vi "TDMS Playback Functional.vi"(1 "Scale Factor Linear":dbl=1.1934598400763813e-07, 4 "IQ Swap Enabled":bool=TRUE, 5 "IQ Rate (S/s)":dbl=25000000.0 format="%#_3p", 6 "pre filter gain":dbl, 7 "channel name (iq/qi)":string="qi", 8 "error in":errorcluster={"status"=FALSE, "code"=373504, "source"="niRFSG Close.vi<ERR>DSP overflow detected. The output waveform was clipped. Reduce the Arb Pre-filter Gain to eliminate overflow."}, 9 "Output Power (dBm)":dbl=10.0 format="%#_3p", 10 "Carrier (Hz)":dbl=3550000000.0 format="%#_3p", 11 "Path":path=path "D:/FOUO/1RDR1P1RDR3.tdms.tdms") -> (0 "error out":errorcluster={"status"=FALSE, "code"=373504, "source"="niRFSG Close.vi<ERR>DSP overflow detected. The output waveform was clipped. Reduce the Arb Pre-filter Gain to eliminate overflow."}, 2 "Playback Progress":i32(slide)=383 scale=-1.0..536.0)   [LabVIEW 2017]
uses:
  <instrlib>/niRFSG/niRFSG.llb/niRFSG Write Arb Waveform (Complex DBL).vi
  MainVI/GlobalVariableS.vi
  <vilib>/FPGAPlugInAG/Dynamic/niLvFpga_Close_Dynamic.vi
  <vilib>/rvi/interface/nirviCloseFPGA/nirviCloseFPGA.xnode
panel:
  out "result string 2":string="3-19-2018"
  in  "input string":string
  out "20 log (scale Factor_Linear)":dbl=-138.46384380841334
  in  "RF:LO Out Enabled":bool
  out "RF:LO Out Power (dBm)":dbl=-0.06505490226659383
  in  "RF:External Gain (dB)":dbl
  in  "RF:Peak Power Adjustment (dB)":dbl
  out "RF:Peak Envelope Power (dBm) =\nPeak Power Adjustment + Output Power":dbl=10.0
  out "RF:Upconverter:Gain (dB)":dbl=4.739916294852831
  out "samples":u32=769639589
  out "number of pending reads 1":u32=8
  out "empty elements":u32=134217728
  out "dma fullness":u32=48764
  out "number of pending reads 2":u32=1
  out "# of elements in host buffer avail for writing":u32=65536
  out "peak fullness":u32
  out "fullness":u32=65536
  out "Completion Loop":i32=3891
  out "fpga peak":u32(slide)=272 scale=-1.0..65536.0
  in  "Monitor Buffer Fullness":bool=TRUE
  out "file peak":u32(slide)=2 scale=0.0..8.0
  out "host peak":u32(slide)=1024 scale=-1.0..134217728.0
  out "File Read Buffer Fullness":u32(slide)=1 scale=0.0..8.0
  out "DMA Host Buffer Emptiness":u32(slide) scale=-1.0..134217728.0
  out "DMA FPGA Buffer Emptiness":u32(slide)=424 scale=-1.0..65536.0
  out "Underflow Detected":bool
  in  "stop button":bool
  in  "Read Block Size (MB)":u32=32 caption="Chunk Size (S)" format="%.0f MB"
  in  "chunks":u32=16 caption="DMA Host Buffer Depth (Blocks)" format="%.0p"
  in  "VST Resource":string="VST"
  # "Config"
  # "Status"
  # "File"
  # "Current"
  # "10/11/2017: +8.57dBm gave -7.23dBm output of the highest peak \n==> Compensate and used Output Power of +8.57+0.24=\n+8.8 dBM to get -7dBm"
  # "Peak"
  # "Current"
  # "Peak"
  # "10/19/2017: +8.8dBm gave -6.44dBm output of the highest peak \n==> Compensate and used Output Power of +8.8-0.47=\n+8.33 dBM to get -7dBm"
  # "RF"
  # "Current"
  # "Peak"
  # "10/19/2017: AutoCal \n==> +8.33 dBm gave -7.22dBm output of the highest peak \n==> Compensate and used Output Power of +8.33+0.22=\n+8.55 dBM to get -7dBm"
  # "Before any other signal processing. \nReduce it to prevent overflow in the AWG interpolation filters. \nSaturates at 7 dB."
  # "After filtering. \nAdjust the output power while keeping the analog path fixed."
  # "Compensate for any Attenuation/Amplification \nbetween Output and DUT"
  # "Refers to PAPR, only used in PEAK Power type.\nIt adds up to Output Power."
  # "20log(1.1534E-6)=  -118.76 dBW\n-118.76 dBW + Correction Factor = -16 dBW \nCorrection Factor = 104.6 dBW"
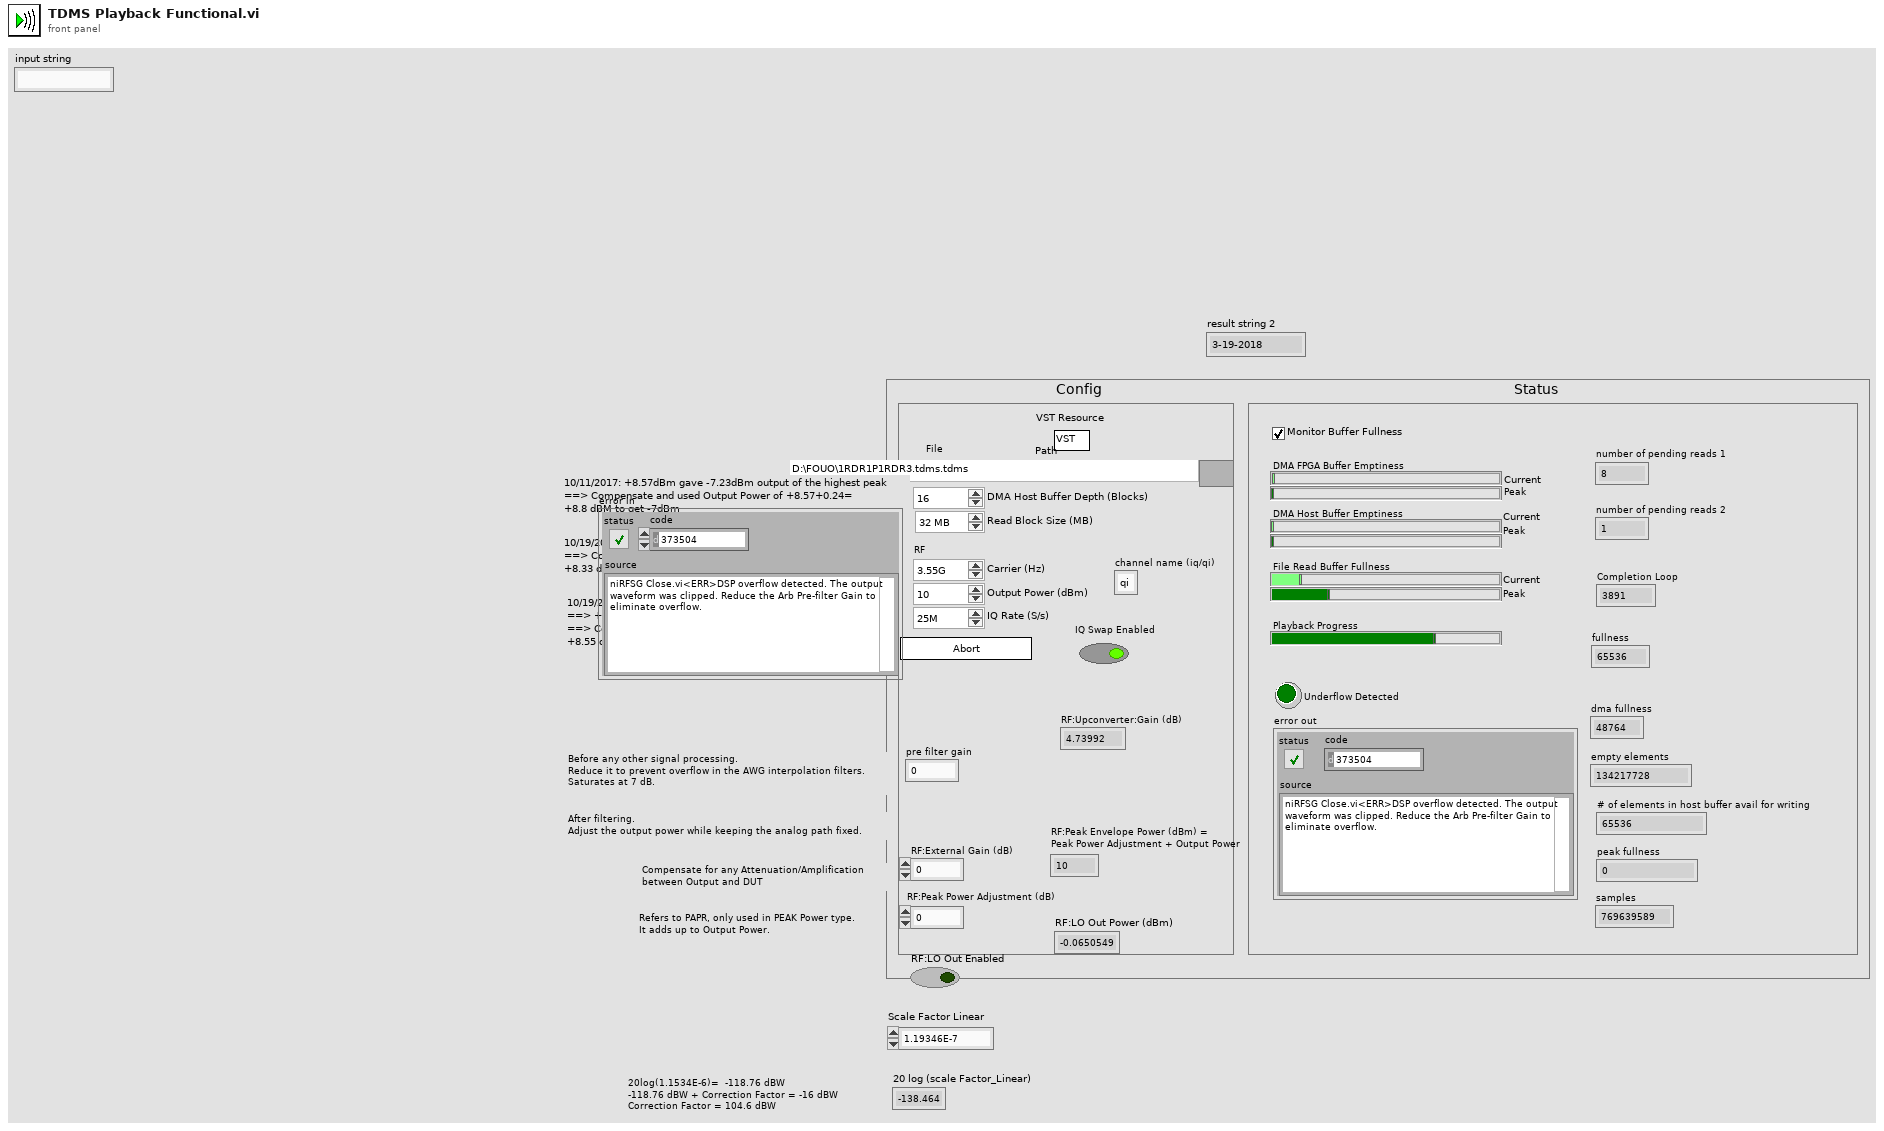
[diagram p1: front panel]
types:
  T1 = enum16{"open", "open or create", "create or replace", "create", "open (read-only)"}
  T2 = cluster{"underflow":bool, "underflows":u32, "samples":u32}
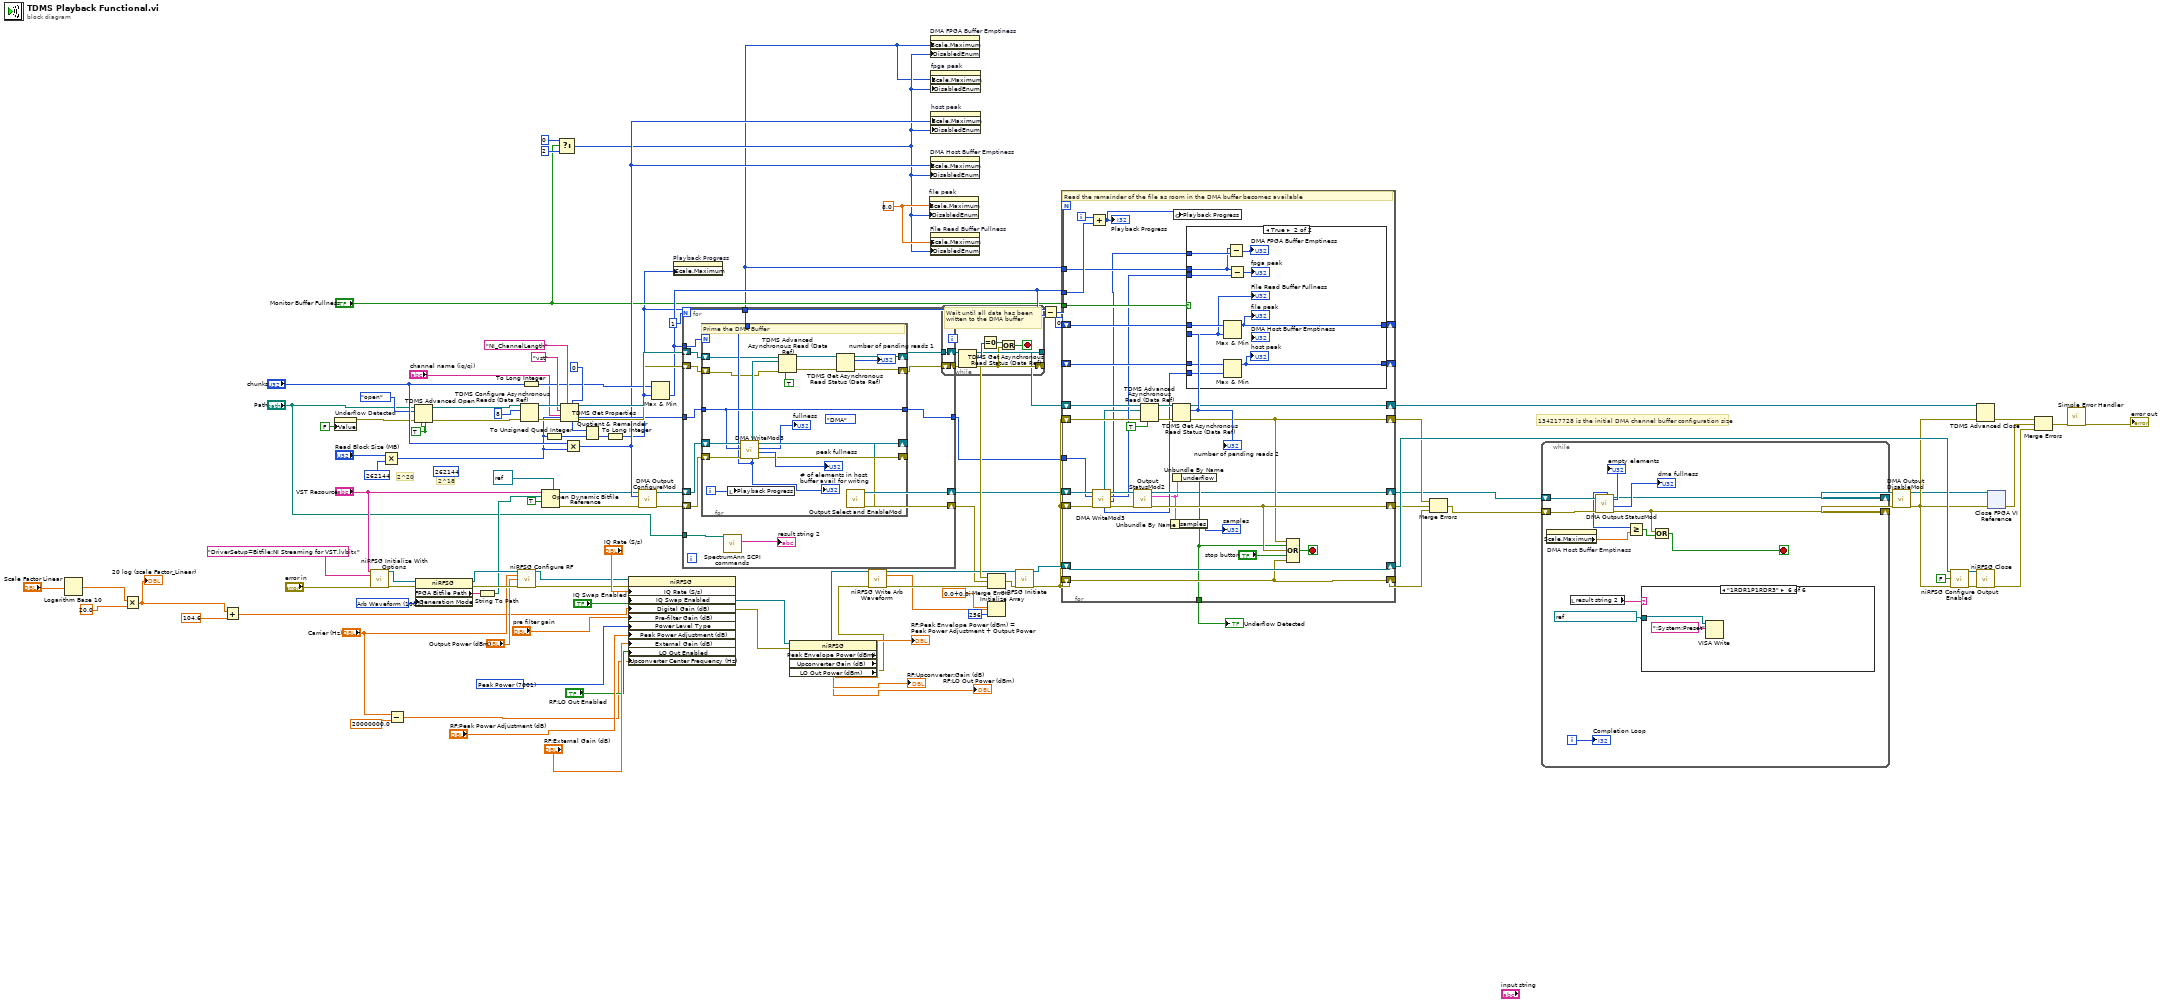
[diagram p0: block diagram]
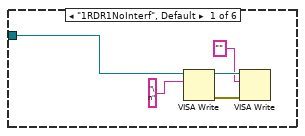
[diagram p3: hidden frame]
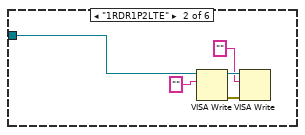
[diagram p4: hidden frame]
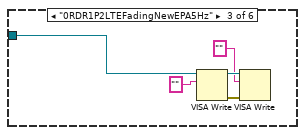
[diagram p5: hidden frame]
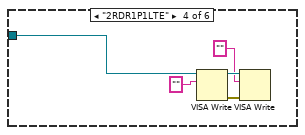
[diagram p6: hidden frame]
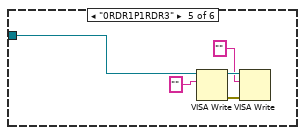
[diagram p7: hidden frame]
diagram:
  w27 = 7001 items=["Average Power"=7000, "Peak Power"=7001] ("RF:Power Level Type")
  (unwired) u32 262144 ("y")
  w51 = 8.0 ("Scale.Range:Maximum")
  w15 = TRUE ("disable buffering? (T)")
  w105 = 1001 items=["CW"=1000, "Arb Waveform"=1001, "Script"=1002] ("Arb:Generation Mode")
  # "134217728 is the initial DMA channel buffer configuration size"
  # "2^20"
  # "2^18"
  n1 = Logarithm Base 10(1:"Scale Factor Linear") -> (0:w9:dbl)
  n2 = Multiply(x=w9, y=20.0) -> (x*y=w8:dbl)
  "20 log (scale Factor_Linear)" <- w8
  n3 = Add(x=w8, y=104.6) -> (x+y=w4:dbl)
  n4 = property on="Underflow Detected" class="Bool (strict)"("Value"=FALSE ("Underflow Detected")) -> (error out=w49:errorcluster)  [unwired: 2 in, 1 out]
  n5 = call <instrlib>:"niRFSG Initialize With Options.vi"("resource name"="VST Resource", "option string"="DriverSetup=Bitfile:NI Streaming for VST.lvbitx", "error in"="error in") -> ("instrument handle"=w110:refnum<k15>, "error out"=w111:errorcluster)  [unwired: 11 in]
  n6 = Multiply(x="Read Block Size (MB)", y=u32 262144) -> (x*y=w59:u32)
  n7 = Subtract(x="Carrier (Hz)", y=20000000.0) -> (x-y=w10:dbl)
  n8 = TDMS Advanced Open(4:w15, 6:w15, 8:w49, 10:T1."open" ("operation (0:open)"), 11:"Path") -> (0:w101:errorcluster, 3:w100:refnum<k34>)  [unwired: 1 out]
  n9 = property class="niRFSG"(reference=w110, error in=w111, "Generation Mode"=w105) -> (reference out=w108:refnum<k15>, error out=w109:errorcluster, "FPGA Bitfile Path"=w107:string)
  n10 = String To Path(string=w107) -> (path=w39:path)
  n11 = call <instrlib>:"niRFSG Configure RF.vi"("instrument handle"=w108, "frequency (Hz)"="Carrier (Hz)", "power level (dBm)"="Output Power (dBm)", "error in"=w109) -> ("instrument handle out"=w26:refnum<k15>, "error out"=w25:errorcluster)  [unwired: 10 in]
  n12 = TDMS Configure Asynchronous Reads (Data Ref)(8:w101, 10:u32 8 ("max asynchronous reads (4)"), 11:w100) -> (0:w90:errorcluster, 3:w91:refnum<k34>)  [unwired: 2 in]
  n13 = To Long Integer(number="chunks") -> (32bit integer=w84:i32)
  n14 = Open Dynamic Bitfile Reference(0:"VST Resource", 1:w39, 2:TRUE ("Run When Loaded"), 4:refnum<k20> refnum ("Type")) -> (5:w30:refnum<k20>, 8:w29:errorcluster)  [unwired: 1 in]
  n15 = To Unsigned Quad Integer(1:w59) -> (0:w62:u64)
  n16 = Select(t=0, s="Monitor Buffer Fullness", f=2) -> (s? t:f=w45:i32)
  n17 = TDMS Get Properties(5:u64 0, 7:"NI_ChannelLength" ("property name"), 8:w90, 9:"channel name (iq/qi)", 10:"vst" ("group name"), 11:w91) -> (0:w88:errorcluster, 3:w89:refnum<k34>, 4:w67:u64)  [unwired: 3 out]
  n18 = Multiply(x="chunks", y=w59) -> (x*y=w57:u32)
  n19 = Quotient & Remainder(x=w67, y=w62) -> (floor(x/y)=w66:u64)  [unwired: 1 out]
  n20 = To Long Integer(number=w66) -> (32bit integer=w52:i32)
  n21 = property class="niRFSG"(reference=w26, error in=w25, "IQ Rate (S/s)"="IQ Rate (S/s)", "IQ Swap Enabled"="IQ Swap Enabled", "Digital Gain (dB)"=w4, "Pre-filter Gain (dB)"="pre filter gain", "Power Level Type"=w27, "Peak Power Adjustment (dB)"="RF:Peak Power Adjustment (dB)", "External Gain (dB)"="RF:External Gain (dB)", "LO Out Enabled"="RF:LO Out Enabled", "Upconverter Center Frequency (Hz)"=w10) -> (reference out=w22:refnum<k15>, error out=w20:errorcluster)
  n22 = call "DMA Output ConfigureMod.vi"("error in (no error)"=w29, "depth"=w57, "Refnum in"=w30) -> ("error out"=w47:errorcluster, "Refnum out"=w46:refnum<k20>)  [unwired: 7 in]
  n23 = Max & Min(x=w84, y=w52) -> (min(x,y)=w61:i32)  [unwired: 1 out]
  n24 = property on="Playback Progress" class="Slide (strict)"("Scale.Maximum"=w52) -> ()  [unwired: 2 in, 2 out]
  n25 = for {
    N: 1 -> [_]
    tunnel: w61 -> [w124]
    tunnel: w59 -> [w123]
    tunnel: [w119] -> w44
    tunnel: [w117] -> w38
    shift-right: [w128] -> w99
    shift-left: w89 -> [w126]
    shift-right: [w127] -> w98
    shift-left: w88 -> [w125]
    shift-right: [w122] -> w48
    shift-left: w47 -> [w121]
    shift-right: [w118] -> w41
    shift-left: w46 -> [w120]
    tunnel: "Path" -> [w113]
    n26 = for {
      N: w124 -> [_]
      shift-right: [w133] -> w127
      shift-left: w125 -> [w129]
      shift-right: [w136] -> w116
      shift-left: w121 -> [w145]
      shift-right: [w132] -> w128
      shift-left: w126 -> [w130]
      shift-right: [w144] -> w115
      shift-left: w120 -> [w146]
      tunnel: w123 -> [w143]
      tunnel: [w143] -> w117
      tunnel: [w141] -> w119
      i -> [w142]
      (unwired) enum16{"none", "DMA", "local", "P2P", "DIO"}."DMA" ("stream select")
      # "Prime the DMA Buffer"
      n27 = local write "Playback Progress"(w142) -> ()
      n28 = call "DMA WriteMod3.vi"("error in (no error)"=w145, "number of elements"=w143, "Refnum in"=w146) -> ("error out"=w136:errorcluster, "peak fullness"=→"peak fullness":u32, "fullness"=→"fullness":u32, "Refnum out"=w144:refnum<k20>, "empty elements remaining"=w141:u32, "Write Region Reference"=w140:refnum<data-value>)  [unwired: 3 in]
      "# of elements in host buffer avail for writing" <- w141
      n29 = TDMS Advanced Asynchronous Read (Data Ref)(6:TRUE ("auto delete reference? (T)"), 8:w129, 10:w140, 11:w130) -> (0:w134:errorcluster, 3:w135:refnum<k34>)  [unwired: 1 out]
      n30 = TDMS Get Asynchronous Read Status (Data Ref)(8:w134, 11:w135) -> (0:w133:errorcluster, 2:→"number of pending reads 1":u32, 3:w132:refnum<k34>)
    }
    n31 = call "SpectrumAnn SCPI commands.vi"("Path"=w113) -> ("result string"=→"result string 2":string)  [unwired: 8 in, 2 out]
    n32 = call "Output Select and EnableMod.vi"("error in (no error)"=w116, "Refnum in"=w115) -> ("error out"=w122:errorcluster, "Refnum out"=w118:refnum<k20>)  [unwired: 8 in]
  }
  n33 = property class="niRFSG"(reference=w22, error in=w20) -> (reference out=w21:refnum<k15>, error out=w19:errorcluster, "Peak Envelope Power (dBm)"=→"RF:Peak Envelope Power (dBm) =\nPeak Power Adjustment + Output Power":dbl, "Upconverter Gain (dB)"=→"RF:Upconverter:Gain (dB)":dbl, "LO Out Power (dBm)"=→"RF:LO Out Power (dBm)":dbl)
  n34 = property on="file peak" class="Slide (strict)"("Scale.Maximum"=w51, "DisabledEnum"=w45) -> ()  [unwired: 2 in, 2 out]
  n35 = property on="DMA FPGA Buffer Emptiness" class="Slide (strict)"("Scale.Maximum"=w44, "DisabledEnum"=w45) -> ()  [unwired: 2 in, 2 out]
  n36 = property on="DMA Host Buffer Emptiness" class="Slide (strict)"("Scale.Maximum"=w57, "DisabledEnum"=w45) -> ()  [unwired: 2 in, 2 out]
  n37 = property on="File Read Buffer Fullness" class="Slide (strict)"("Scale.Maximum"=w51, "DisabledEnum"=w45) -> ()  [unwired: 2 in, 2 out]
  n38 = property on="fpga peak" class="Slide (strict)"("Scale.Maximum"=w44, "DisabledEnum"=w45) -> ()  [unwired: 2 in, 2 out]
  n39 = property on="host peak" class="Slide (strict)"("Scale.Maximum"=w57, "DisabledEnum"=w45) -> ()  [unwired: 2 in, 2 out]
  n40 = while {
    tunnel: w99 -> [w152]
    shift-right: [w148] -> w95
    shift-left: w98 -> [w153]
    tunnel: [w150] -> w94
    stop <- w149 stop-if-true
    # "Wait until all data has been written to the DMA buffer"
    n41 = TDMS Get Asynchronous Read Status (Data Ref)(8:w153, 11:w152) -> (0:w148:errorcluster, 2:w151:u32, 3:w150:refnum<k34>)
    n42 = Equal To 0?(x=w151) -> (x = 0?=w147:bool)
    n43 = Or(x=w147, y=w148) -> (x .or. y?=w149:bool)
  }
  n44 = Initialize Array(cdb 0.0+0.0i ("element"), 256 ("dimension size")) -> (w35:cdb[])
  n45 = call-poly <instrlib>:"niRFSG Write Arb Waveform.vi"("instrument handle"=w21, "waveform data"=w35, "error in"=w19) -> ("instrument handle out"=w82:refnum<k15>, "error out"=w81:errorcluster)  [unwired: 11 in]
  n46 = Merge Errors(w95, w48, w81) -> (w97:errorcluster)
  n47 = call <instrlib>:"niRFSG Initiate.vi"("instrument handle"=w82, "error in"=w97) -> ("instrument handle out"=w96:refnum<k15>, "error out"=w83:errorcluster)  [unwired: 12 in]
  n48 = Subtract(x=w52, y=w61) -> (x-y=w60:i32)
  n49 = for {
    N: w60 -> [_]
    shift-right: [w187] -> w70
    shift-left: w83 -> [w187]
    shift-right: [w168] -> w71
    shift-left: w83 -> [w175]
    shift-right: [w171] -> w72
    shift-left: w83 -> [w176]
    shift-right: [w167] -> w92
    shift-left: w94 -> [w174]
    shift-right: [w188] -> w78
    shift-left: w96 -> [w188]
    tunnel: w61 -> [w184]
    tunnel: w38 -> [w161]
    tunnel: [w165] -> w58
    shift-right: [w181] -> _
    shift-left: u32 0 -> [w180]
    shift-right: [w179] -> _
    shift-left: _ -> [w178]
    tunnel: "Monitor Buffer Fullness" -> [w177]
    tunnel: w44 -> [w164]
    shift-right: [w160] -> w40
    shift-left: w41 -> [w162]
    i -> [w183]
    stop <- w185 stop-if-true
    # "Read the remainder of the file as room in the DMA buffer becomes available"
    n50 = Add(x=w183, y=w184) -> (x+y=w154:i32)
    "Playback Progress" <- w154
    n51 = call "DMA WriteMod3.vi"("error in (no error)"=w176, "number of elements"=w161, "Refnum in"=w162) -> ("error out"=w172:errorcluster, "peak fullness"=w157:u32, "fullness"=w166:u32, "Refnum out"=w173:refnum<k20>, "empty elements remaining"=w159:u32, "Write Region Reference"=w158:refnum<data-value>)  [unwired: 3 in]
    n52 = call "Output StatusMod2.vi"("error in (no error)"=w172, "Refnum in"=w173) -> ("error out"=w171:errorcluster, "status"=w156:T2, "Refnum out"=w160:refnum<k20>)  [unwired: 7 in]
    n53 = TDMS Advanced Asynchronous Read (Data Ref)(6:TRUE ("auto delete reference? (T)"), 8:w175, 10:w158, 11:w174) -> (0:w170:errorcluster, 3:w169:refnum<k34>)  [unwired: 1 out]
    n54 = Unbundle By Name(w156) -> ("samples"=→"samples":u32)
    n55 = TDMS Get Asynchronous Read Status (Data Ref)(8:w170, 11:w169) -> (0:w168:errorcluster, 2:w182:u32, 3:w167:refnum<k34>)
    "number of pending reads 2" <- w182
    n56 = Unbundle By Name(w156) -> ("underflow"=w165:bool)
    n57 = global write "GlobalVariableS.vi" "Playback Progress"(w154) -> ()
    n58 = case shown="True" w177 {
      tunnel: w182 -> [_ w198]
      tunnel: [_ w196] -> w181
      tunnel: w180 -> [_ w199]
      tunnel: [_ w195] -> w179
      tunnel: w178 -> [_ w197]
      tunnel: w157 -> [_ w191]
      tunnel: w166 -> [_ w193]
      tunnel: w159 -> [_ w194]
      tunnel: w164 -> [_ w190]
      frame False {
      }
      frame True {
        n59 = Max & Min(x=w199, y=w198) -> (max(x,y)=w196:u32)  [unwired: 1 out]
        "file peak" <- w196
        n60 = Max & Min(x=w197, y=w194) -> (max(x,y)=w195:u32)  [unwired: 1 out]
        "host peak" <- w195
        n61 = Subtract(x=w190, y=w191) -> (x-y=→"DMA FPGA Buffer Emptiness":u32)
        n62 = Subtract(x=w190, y=w193) -> (x-y=→"fpga peak":u32)
        "File Read Buffer Fullness" <- w198
      }
    }
    n63 = Compound Arithmetic op=OR(w168, w165, w171, "stop button", w187) -> (w185:bool)
  }
  "Underflow Detected" <- w58
  n64 = Merge Errors(w71, w72, w70) -> (w93:errorcluster)
  n65 = while {
    shift-right: [w207] -> w80
    shift-left: w93 -> [w211]
    shift-right: [w202] -> w79
    shift-left: w40 -> [w210]
    i -> [w209]
    stop <- w208 stop-if-true
    n66 = property on="DMA Host Buffer Emptiness" class="Slide (strict)"() -> ("Scale.Maximum"=w203:dbl)  [unwired: 2 in, 2 out]
    n67 = local read "result string 2"() -> (w200:string)
    n68 = call "DMA Output StatusMod.vi"("error in (no error)"=w211, "Refnum in"=w210) -> ("error out"=w207:errorcluster, "dma fullness"=→"dma fullness":u32, "Refnum out"=w202:refnum<k20>, "empty elements"=w204:u32)  [unwired: 5 in, 1 out]
    "empty elements" <- w204
    n69 = Greater Or Equal?(x=w204, y=w203) -> (x >= y?=w206:bool)
    n70 = case shown="\"1RDR1P1RDR3\"" w200 {
      tunnel: refnum<visa-resource-name> "SpecAnn-9010A-20100" ("VISA resource name") -> [w212 w217 w222 w227 w232 w238]
      frame "1RDR1NoInterf", Default {
        n71 = VISA Write(VISA resource name=w212, write buffer="\n") -> (VISA resource name out=w215:refnum<visa-resource-name>, error out=w214:errorcluster)  [unwired: 1 in, 1 out]
        n72 = VISA Write(VISA resource name=w215, write buffer="", error in (no error)=w214) -> ()  [unwired: 3 out]
      }
      frame "1RDR1P2LTE" {
        n73 = VISA Write(VISA resource name=w217, write buffer="") -> (VISA resource name out=w220:refnum<visa-resource-name>, error out=w219:errorcluster)  [unwired: 1 in, 1 out]
        n74 = VISA Write(VISA resource name=w220, write buffer="", error in (no error)=w219) -> ()  [unwired: 3 out]
      }
      frame "0RDR1P2LTEFadingNewEPA5Hz" {
        n75 = VISA Write(VISA resource name=w222, write buffer="") -> (VISA resource name out=w225:refnum<visa-resource-name>, error out=w224:errorcluster)  [unwired: 1 in, 1 out]
        n76 = VISA Write(VISA resource name=w225, write buffer="", error in (no error)=w224) -> ()  [unwired: 3 out]
      }
      frame "2RDR1P1LTE" {
        n77 = VISA Write(VISA resource name=w227, write buffer="") -> (VISA resource name out=w230:refnum<visa-resource-name>, error out=w229:errorcluster)  [unwired: 1 in, 1 out]
        n78 = VISA Write(VISA resource name=w230, write buffer="", error in (no error)=w229) -> ()  [unwired: 3 out]
      }
      frame "0RDR1P1RDR3" {
        n79 = VISA Write(VISA resource name=w232, write buffer="") -> (VISA resource name out=w235:refnum<visa-resource-name>, error out=w234:errorcluster)  [unwired: 1 in, 1 out]
        n80 = VISA Write(VISA resource name=w235, write buffer="", error in (no error)=w234) -> ()  [unwired: 3 out]
      }
      frame "1RDR1P1RDR3" {
        n81 = VISA Write(VISA resource name=w238, write buffer=":System:Preset") -> ()  [unwired: 1 in, 3 out]
      }
    }
    n82 = Compound Arithmetic op=OR(w207, w206) -> (w208:bool)
    "Completion Loop" <- w209
  }
  n83 = call "DMA Output DisableMod.vi"("error in (no error)"=w80, "Refnum in"=w79) -> ("error out"=w32:errorcluster, "Refnum out"=w31:refnum<k20>)  [unwired: 8 in]
  n84 = call <instrlib>:"niRFSG Configure Output Enabled.vi"("instrument handle"=w78, "output enabled"=FALSE, "error in"=w32) -> ("instrument handle out"=w76:refnum<k15>, "error out"=w77:errorcluster)  [unwired: 11 in]
  n85 = TDMS Advanced Close(8:w32, 11:w92) -> (0:w65:errorcluster)  [unwired: 2 in, 1 out]
  n86 = call <instrlib>:"niRFSG Close.vi"("instrument handle"=w76, "error in"=w77) -> ("error out"=w63:errorcluster)  [unwired: 13 in]
  n87 = xnode "Close FPGA VI Reference"("FPGA VI Reference In"=w31, "error in"=w32) -> ("error out"=w64:errorcluster)
  n88 = Merge Errors(w65, w64, w63) -> (w33:errorcluster)
  "error out" <- w33
  n89 = call <vilib>:"Simple Error Handler.vi"("error in (no error)"=w33) -> ()  [unwired: 4 in, 5 out]
